vi "Post-Build Action.vi"(5 "Files Generated by Build":path[](array[path]), 6 "Top Level/Always Included VIs":path[](array[path]), 7 "Destination Path":path, 8 "error in (no error)":errorcluster, 9 "Target Name":string, 10 "Build Specification Name":string, 11 "Project Path":path) -> (0 "error out":errorcluster)   [LabVIEW 2019]
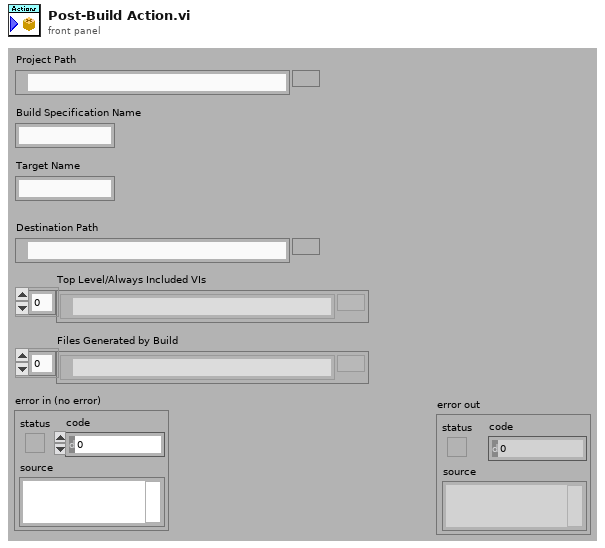
[diagram p1: front panel]
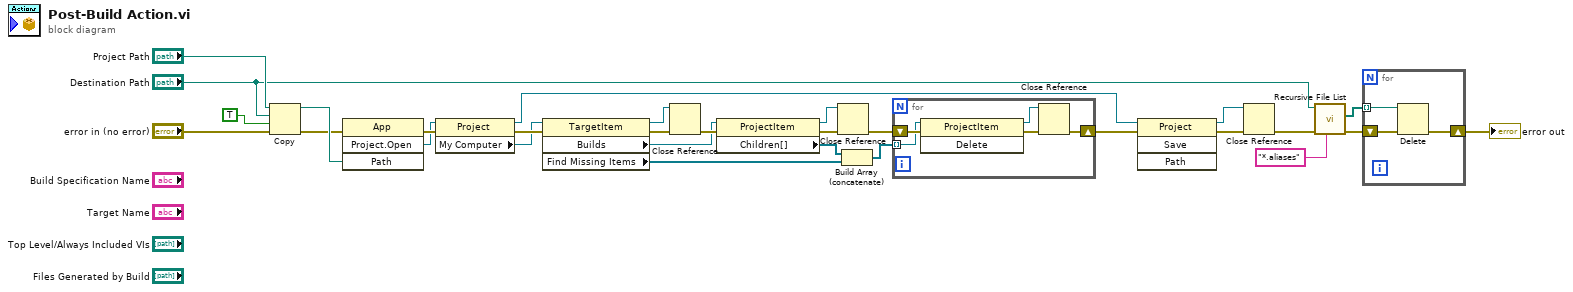
[diagram p0: block diagram]
diagram:
  n1 = Copy(8:"error in (no error)", 9:TRUE ("overwrite (F)"), 10:"Destination Path", 11:"Project Path") -> (0:w22:errorcluster, 3:w28:path)  [unwired: 1 in, 1 out]
  n2 = invoke class="App" method="Project.Open"(error in=w22, "Path"=w28) -> (error out=w25:errorcluster, "Project:Open"=w13:refnum<vi>)  [unwired: 2 in, 2 out]
  n3 = property class="Project"(reference=w13, error in=w25) -> (reference out=w27:refnum<vi>, error out=w26:errorcluster, "My Computer"=w11:refnum<vi>)
  n4 = property class="TargetItem"(reference=w11, error in=w26) -> (reference out=w15:refnum<vi>, error out=w16:errorcluster, "Builds"=w12:refnum<vi>, "Find Missing Items"=w9:refnum<vi>[])
  n5 = Close Reference(reference=w15, error in (no error)=w16) -> (error out=w14:errorcluster)
  n6 = property class="ProjectItem"(reference=w12, error in=w14) -> (reference out=w18:refnum<vi>, error out=w19:errorcluster, "Children[]"=w10:refnum<vi>[])
  n7 = Close Reference(reference=w18, error in (no error)=w19) -> (error out=w17:errorcluster)
  n8 = Build Array (concatenate)(w10, w9) -> (w8:refnum<vi>[])
  n9 = for {
    shift-right: [w31] -> w7
    shift-left: w17 -> [w34]
    tunnel: w8 -> [w33] mode=indexing
    n10 = invoke class="ProjectItem" method="Delete"(reference=w33, error in=w34) -> (reference out=w30:refnum<vi>, error out=w32:errorcluster)  [unwired: 1 in, 1 out]
    n11 = Close Reference(reference=w30, error in (no error)=w32) -> (error out=w31:errorcluster)
  }
  n12 = invoke class="Project" method="Save"(reference=w27, error in=w7) -> (reference out=w20:refnum<vi>, error out=w21:errorcluster)  [unwired: 2 in, 2 out]
  n13 = Close Reference(reference=w20, error in (no error)=w21) -> (error out=w5:errorcluster)
  n14 = call <vilib>:"Recursive File List.vi"("pattern"="*.aliases", "error in (no error)"=w5, "Folder Path"="Destination Path") -> ("error out"=w3:errorcluster, "All Files in Dir"=w1:path[])  [unwired: 4 in, 3 out]
  n15 = for {
    shift-right: [w35] -> w2
    shift-left: w3 -> [w37]
    tunnel: w1 -> [w36] mode=indexing
    n16 = Delete(path (use dialog)=w36, error in=w37) -> (error out=w35:errorcluster)  [unwired: 3 in, 2 out]
  }
  "error out" <- w2
